vi "Get Block Size.vi"(8 "error in":errorcluster, 11 "Block Upload Initiate in":refnum<class "Block Upload Initiate Transfer.lvclass">) -> (0 "error out":errorcluster, 2 "Block Size":u8=16, 3 "Block Upload Initiate out":refnum<class "Block Upload Initiate Transfer.lvclass">)   [LabVIEW 2020, in "CANopen.lvlib" / "SDO Manager.lvlib" / "Block Upload Initiate Transfer.lvclass"]
uses:
  Block Upload Initiate Transfer.lvclass
  Block Upload Initiate Transfer.lvclass/Block Upload Initiate Transfer.ctl
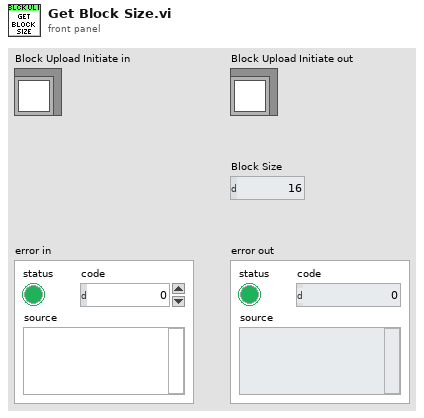
[diagram p1: front panel]
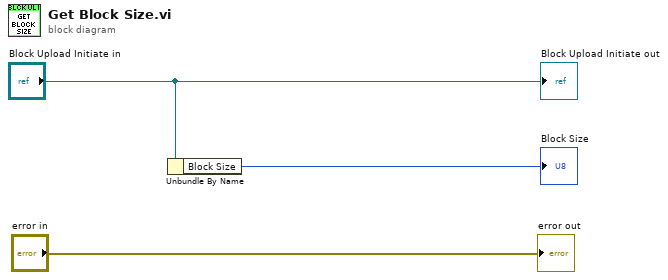
[diagram p0: block diagram]
diagram:
  n1 = Unbundle By Name("Block Upload Initiate in") -> ("Block Size"=→"Block Size":u8)
  "error out" <- "error in"
  "Block Upload Initiate out" <- "Block Upload Initiate in"
